vi "6-18-19-data.vi"() -> ()   [LabVIEW 2016]
uses:
  <vilib>/Analysis/baseanly.llb/Mean (DBL).vi
  <userlib>/Levylab/LV to ITX/LVtoITX.lvclass
  <vilib>/Analysis/NI_AALBase.lvlib
  <vilib>/Analysis/NI_AALPro.lvlib
panel:
  in  "Path":path=path "P:/Users1/Aaron Greenberg/SA40060G.20190618.000003.dat"
  out "output cluster":cluster{dbl[], dbl[], dbl[], dbl[]}
  out "Temp vs Time":cluster{dbl[], dbl[]}(graph)
  out "Time vs Temp":cluster{dbl[], dbl[]}(graph)
  out "G4T Vs Temp":cluster{"Data":dbl[], "Data":dbl[]}[](graph)
  out "G2T Vs Temp":cluster{"Data":dbl[], "Data":dbl[]}[](graph)
  out "Linear Fit":cluster{dbl[], "Best Exponential Fit":dbl[]}[](graph)
  out "Full Data":cluster{dbl[], dbl[]}[](graph)
  in  "header length":i32=11
  out "Comments":string
  out "Wavenames":string[](array[string])
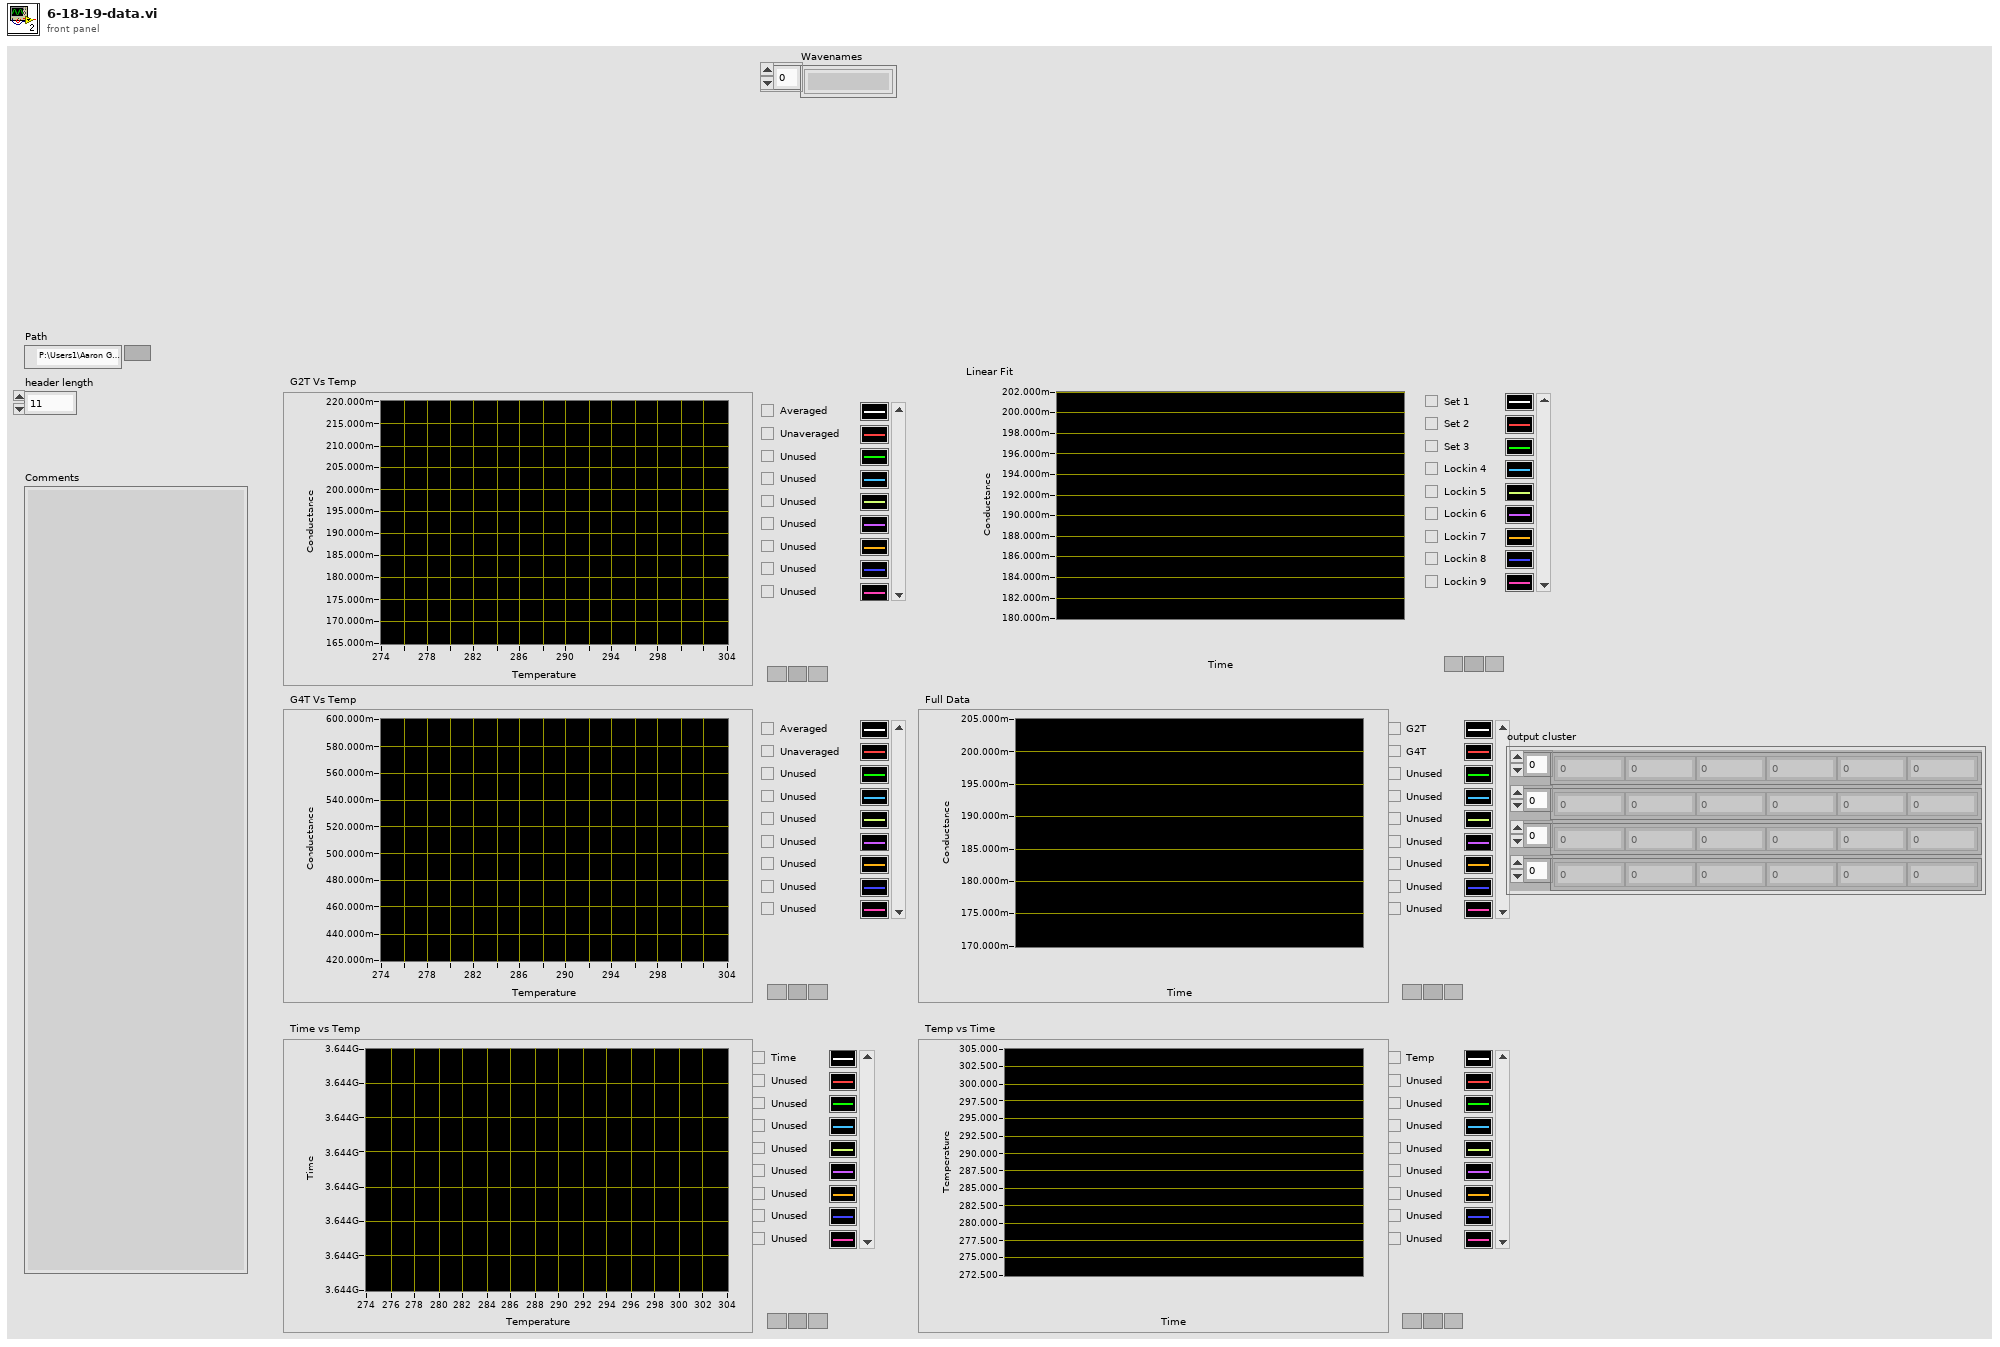
[diagram p1: front panel]
types:
  T1 = cluster{"slope min":dbl, "slope max":dbl, "intercept min":dbl, "intercept max":dbl}
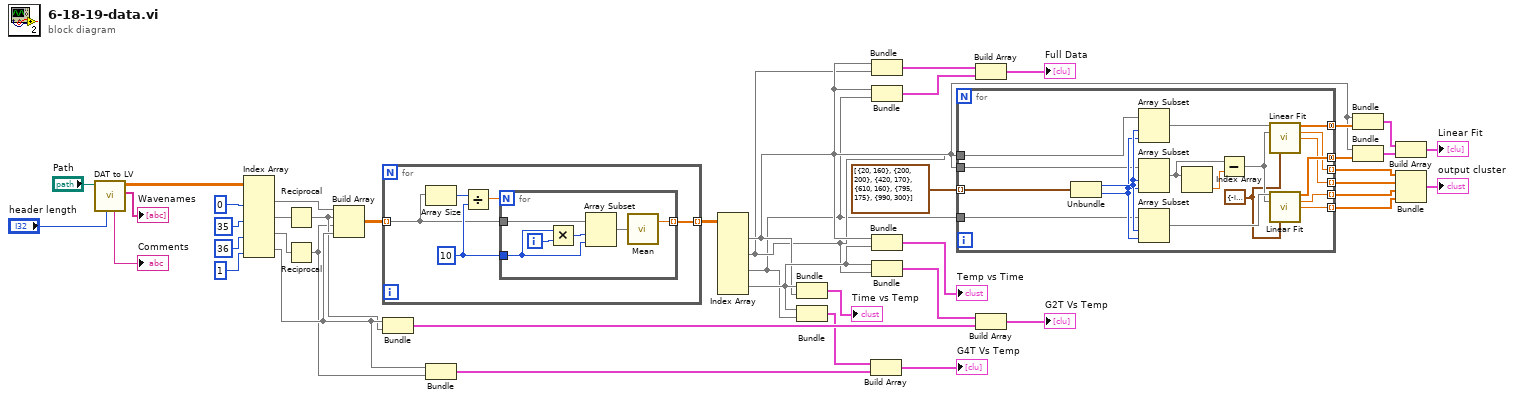
[diagram p0: block diagram]
diagram:
  n1 = call <userlib>:"DAT to LV.vi"("header length"="header length", "File Path"="Path") -> ("Wavenames"=→"Wavenames":string[], "Data"=w41:dbl[][], "Comments"=→"Comments":string)  [unwired: 6 in, 1 out]
  n2 = Index Array(array=w41, index (col) #1=0 ("disabled index (col)"), index (col) #2=35 ("index (col)"), index (col) #3=36 ("index (col)"), index (col) #4=1 ("index (col)")) -> (element #1=w10:dbl[], element #2=w4:dbl[], element #3=w2:dbl[], element #4=w9:dbl[])  [unwired: 4 in]
  n3 = Reciprocal(x=w4) -> (1/x=w3:dbl[])
  n4 = Reciprocal(x=w2) -> (1/x=w1:dbl[])
  n5 = Build Array(w10, w3, w1, w9) -> (w37:dbl[][])
  n6 = for {
    tunnel: w37 -> [w45] mode=indexing
    tunnel: [w44] -> w36 mode=indexing
    w46 = 10 ("x")
    n7 = Array Size(array=w45) -> (size(s)=w48:i32)
    n8 = Divide(x=w48, y=w46) -> (x/y=w47:dbl)
    n9 = for {
      N: w47 -> [_]
      tunnel: w46 -> [w52]
      tunnel: [w51] -> w44 mode=indexing
      tunnel: w45 -> [w50]
      i -> [w54]
      n10 = Multiply(x=w52, y=w54) -> (x*y=w53:i32)
      n11 = Array Subset(array=w50, index=w53, length=w52) -> (w49:dbl[])
      n12 = call-poly <vilib>:"Mean.vi"("X"=w49) -> ("mean"=w51:dbl)  [unwired: 1 out]
    }
  }
  n13 = Bundle("Data"=w9, w3) -> (w22:cluster{"Data":dbl[], dbl[]})  [unwired: 1 in]
  n14 = Bundle("Data"=w9, w1) -> (w21:cluster{"Data":dbl[], dbl[]})  [unwired: 1 in]
  n15 = Index Array(array=w36) -> (element #1=w15:dbl[], element #2=w13:dbl[], element #3=w12:dbl[], element #4=w43:dbl[])  [unwired: 8 in]
  n16 = Bundle(w43, w15) -> (→"Time vs Temp":cluster{dbl[], dbl[]})  [unwired: 1 in]
  n17 = Bundle(w43, w12) -> (w20:cluster{dbl[], dbl[]})  [unwired: 1 in]
  n18 = Build Array(w20, w21) -> (→"G4T Vs Temp":cluster{"Data":dbl[], dbl[]}[])
  n19 = Bundle(w15, w13) -> (w35:cluster{dbl[], dbl[]})  [unwired: 1 in]
  n20 = Bundle(w15, w12) -> (w34:cluster{dbl[], dbl[]})  [unwired: 1 in]
  n21 = Bundle(w15, w43) -> (→"Temp vs Time":cluster{dbl[], dbl[]})  [unwired: 1 in]
  n22 = Bundle(w43, w13) -> (w19:cluster{dbl[], dbl[]})  [unwired: 1 in]
  n23 = for {
    tunnel: cluster{i32, i32}[] [{20, 160}, {200, 200}, {420, 170}, {610, 160}, {795, 175}, {990, 300}] -> [w72] mode=indexing
    tunnel: w15 -> [w69]
    tunnel: w13 -> [w68]
    tunnel: w12 -> [w67]
    tunnel: [w64] -> w28 mode=concatenating
    tunnel: [w63] -> w27 mode=concatenating
    tunnel: [w59] -> w8 mode=indexing
    tunnel: [w58] -> w24 mode=indexing
    tunnel: [w57] -> w7 mode=indexing
    tunnel: [w56] -> w6 mode=indexing
    w55 = T1 {"slope min"=-inf, "slope max"=inf, "intercept min"=-inf, "intercept max"=inf} ("parameter bounds")
    n24 = Unbundle(w72) -> (w71:i32, w70:i32)
    n25 = Array Subset(array=w68, index=w71, length=w70) -> (w66:dbl[])
    n26 = Array Subset(array=w69, index=w71, length=w70) -> (w62:dbl[])
    n27 = Array Subset(array=w67, index=w71, length=w70) -> (w65:dbl[])
    n28 = Index Array(array=w62) -> (element=w61:dbl)  [unwired: 1 in]
    n29 = Subtract(x=w62, y=w61) -> (x-y=w60:dbl[])
    n30 = call <vilib>:"Linear Fit.vi"("Y"=w66, "X"=w60, "parameter bounds"=w55) -> ("Best Linear Fit"=w64:dbl[], "slope"=w59:dbl, "intercept"=w58:dbl)  [unwired: 8 in, 2 out]
    n31 = call <vilib>:"Linear Fit.vi"("Y"=w65, "X"=w60, "parameter bounds"=w55) -> ("Best Linear Fit"=w63:dbl[], "slope"=w57:dbl, "intercept"=w56:dbl)  [unwired: 8 in, 2 out]
  }
  n32 = Build Array(w35, w34) -> (→"Full Data":cluster{dbl[], dbl[]}[])
  n33 = Build Array(w19, w22) -> (→"G2T Vs Temp":cluster{"Data":dbl[], dbl[]}[])
  n34 = Bundle(w15, "Best Linear Fit"=w28) -> (w26:cluster{dbl[], "Best Linear Fit":dbl[]})  [unwired: 1 in]
  n35 = Bundle(w15, "Best Linear Fit"=w27) -> (w25:cluster{dbl[], "Best Linear Fit":dbl[]})  [unwired: 1 in]
  n36 = Build Array(w26, w25) -> (→"Linear Fit":cluster{dbl[], "Best Linear Fit":dbl[]}[])
  n37 = Bundle(w8, w24, w7, w6) -> (→"output cluster":cluster{dbl[], dbl[], dbl[], dbl[]})  [unwired: 1 in]
